vi "V003 - Variable DC Controller + Other Sensors.vi"() -> ()   [LabVIEW 2022 SP3]
uses:
  <vilib>/DAQmx/read.llb/DAQmx Read (Analog 1D DBL NChan 1Samp).vi
  <vilib>/DAQmx/create/channels.llb/DAQmx Create Channel (AI-Voltage-Basic).vi
  <vilib>/DAQmx/miscellaneous.llb/DAQmx Fill In Error Info.vi
panel:
  out "Case 0 Reached 2":bool
  out "Power Appl Ch3":bool
  in  "Appl CH3":bool
  out "Humidity":dbl(knob) scale=60.0..100.0
  out "Temperature":dbl(knob) scale=0.0..40.0
  out "Case 1 reached":bool
  out "CH2 Appl":bool
  in  "Appl CH2":bool
  out "Power On 3":bool
  out "Power On 2":bool
  in  "Turn On CH3":bool
  in  "Turn On CH2":bool
  out "Case 2  Reached":bool
  out "Case 1 Reached":bool
  in  "Numeric Controller Sub":dbl format="%#_1g"
  out "Power On":bool
  in  "Turn On CH1":bool
  out "Case 0 Reached":bool
  out "Connected":bool
  in  "VISA resource name":refnum<visa-resource-name>
  in  "Connect":bool
  in  "Numeric Controller Main":dbl
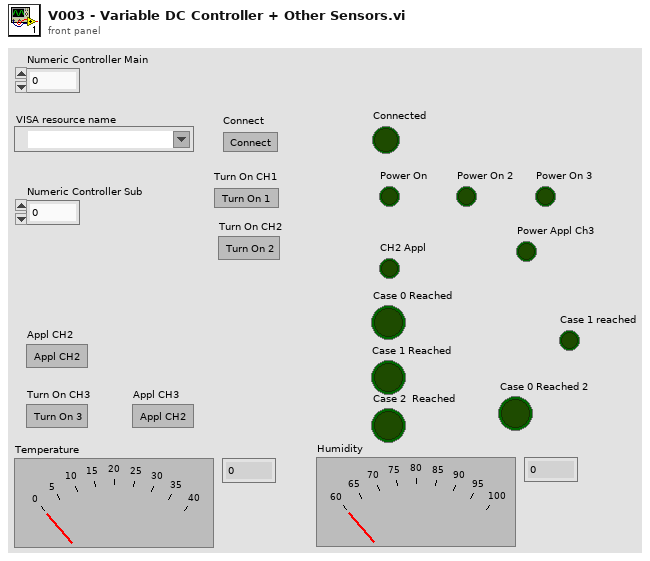
[diagram p1: front panel]
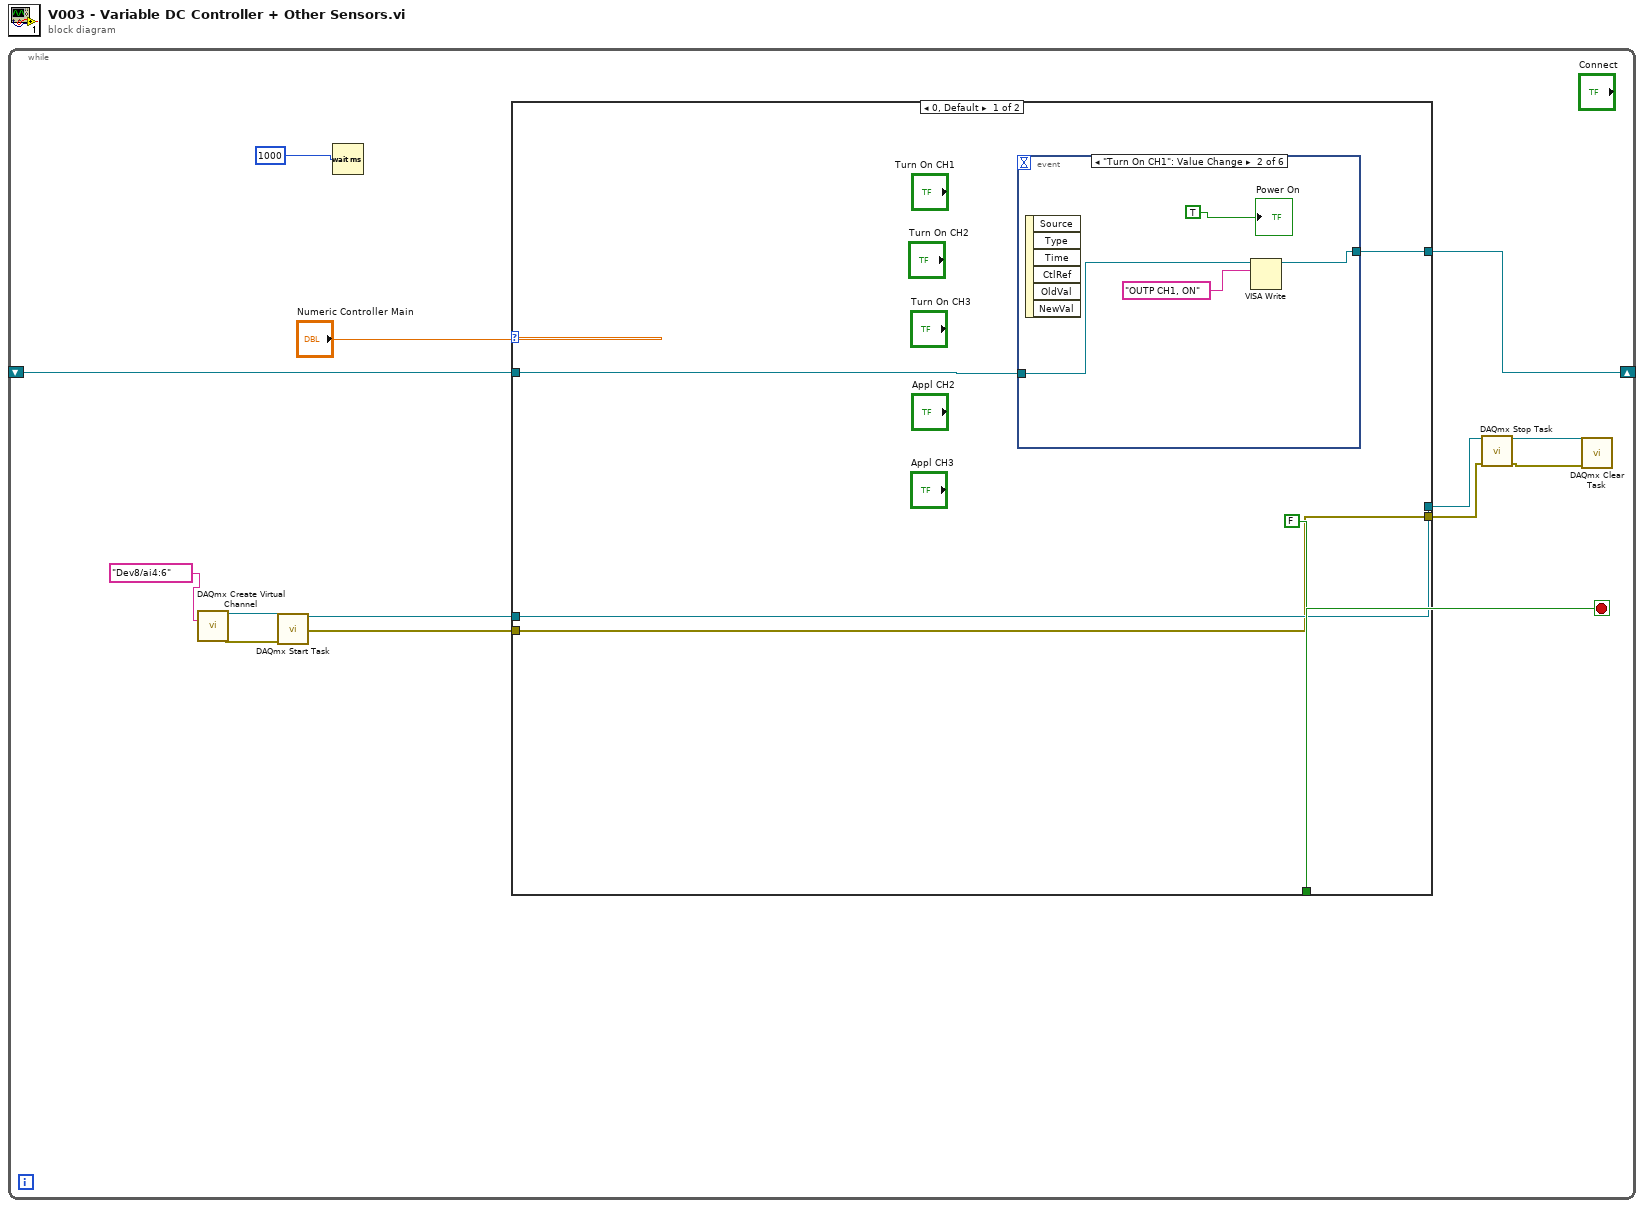
[diagram p0: block diagram]
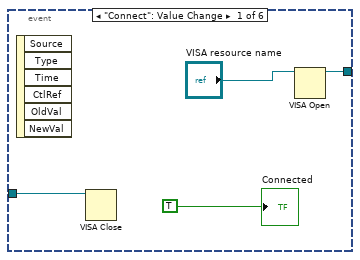
[diagram p2: hidden frame]
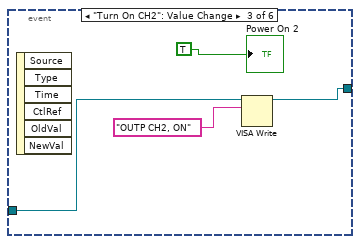
[diagram p3: hidden frame]
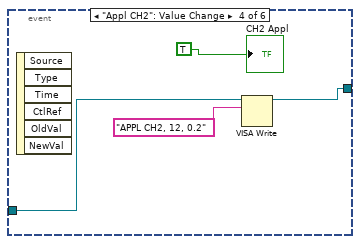
[diagram p4: hidden frame]
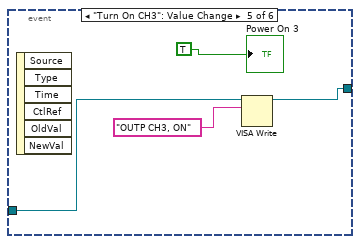
[diagram p5: hidden frame]
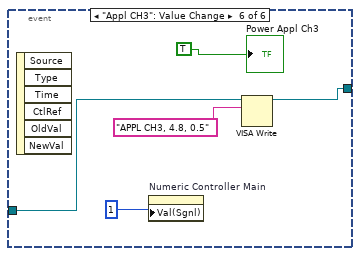
[diagram p6: hidden frame]
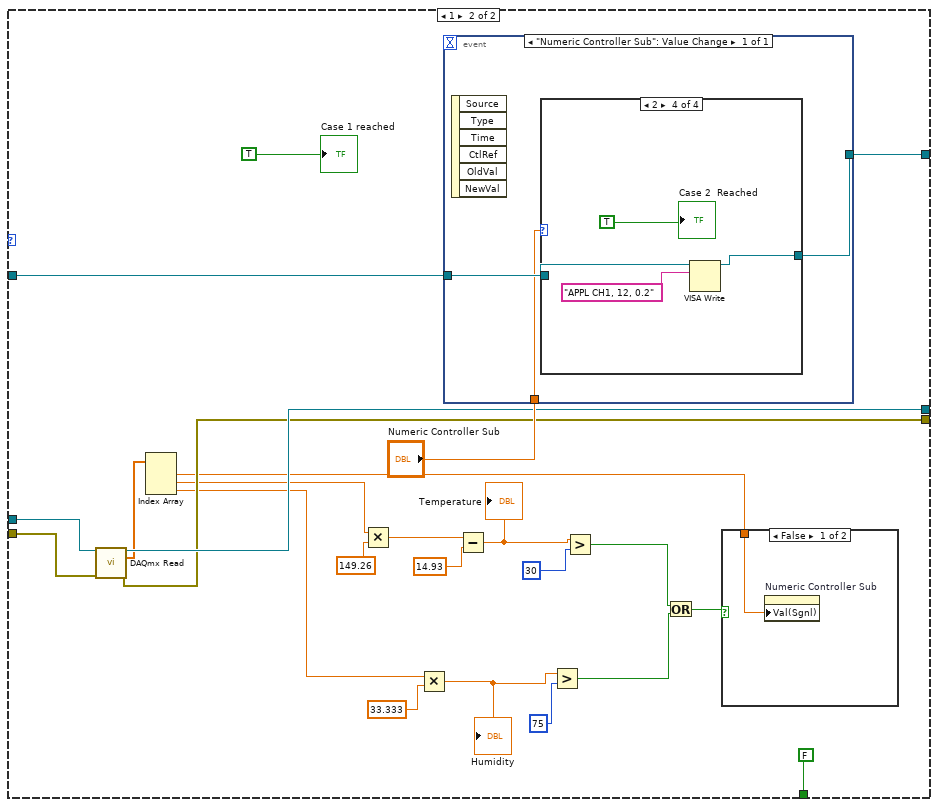
[diagram p7: hidden frame]
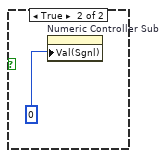
[diagram p8: hidden frame]
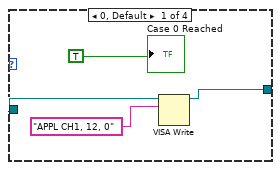
[diagram p9: hidden frame]
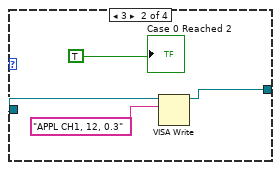
[diagram p10: hidden frame]
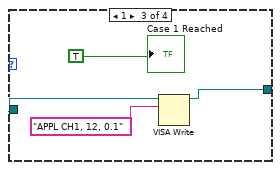
[diagram p11: hidden frame]
diagram:
  n1 = while {
    shift-right: [w13] -> _
    shift-left: _ -> [w14]
    stop <- w12 stop-if-true
    n2 = call-poly <vilib>:"DAQmx Create Virtual Channel.vi"("physical channels"=tag "Dev8/ai4:6") -> ("task out"=w10:refnum<k21>, "error out"=w6:errorcluster)  [unwired: 13 in]
    n3 = call <vilib>:"DAQmx Start Task.vi"("task/channels in"=w10, "error in"=w6) -> ("task out"=w8:refnum<k21>, "error out"=w7:errorcluster)  [unwired: 12 in]
    n4 = Wait (ms)(milliseconds to wait=1000) -> ()  [unwired: 1 out]
    n5 = case shown="0, Default" "Numeric Controller Main" {
      tunnel: w14 -> [w19 w66]
      tunnel: [w18 w67] -> w13
      tunnel: [FALSE FALSE] -> w12
      tunnel: w8 -> [w16 w64]
      tunnel: w7 -> [w15 w62]
      tunnel: [w16 w61] -> w2
      tunnel: [w15 w60] -> w1
      frame 0, Default {
        n6 = event shown="[1] \"Turn On CH1\": Value Change" {
          selector: _ -> [_ _ _ _ _ _]
          dyn-events: _ -> [_ _ _ _ _ _]
          timeout: _ -> [_ _ _ _ _ _]
          tunnel: w19 -> [w23 w26 w30 w34 w38 w43]
          tunnel: [w22 w25 w29 w33 w37 w42] -> w18
          event "Connect": Value Change {
            n7 = event-data() -> ()  [unwired: 1 in, 6 out]
            n8 = VISA Close(VISA resource name=w23) -> ()  [unwired: 1 in, 1 out]
            n9 = VISA Open(VISA resource name="VISA resource name") -> (VISA resource name=w22:refnum<visa-resource-name>)  [unwired: 4 in, 1 out]
            "Connected" <- TRUE
          }
          event "Turn On CH1": Value Change {
            n10 = event-data() -> ()  [unwired: 1 in, 6 out]
            n11 = VISA Write(VISA resource name=w26, write buffer="OUTP CH1, ON") -> (VISA resource name out=w25:refnum<visa-resource-name>)  [unwired: 1 in, 2 out]
            "Power On" <- TRUE
          }
          event "Turn On CH2": Value Change {
            n12 = event-data() -> ()  [unwired: 1 in, 6 out]
            n13 = VISA Write(VISA resource name=w30, write buffer="OUTP CH2, ON") -> (VISA resource name out=w29:refnum<visa-resource-name>)  [unwired: 1 in, 2 out]
            "Power On 2" <- TRUE
          }
          event "Appl CH2": Value Change {
            n14 = event-data() -> ()  [unwired: 1 in, 6 out]
            n15 = VISA Write(VISA resource name=w34, write buffer="APPL CH2, 12, 0.2") -> (VISA resource name out=w33:refnum<visa-resource-name>)  [unwired: 1 in, 2 out]
            "CH2 Appl" <- TRUE
          }
          event "Turn On CH3": Value Change {
            n16 = event-data() -> ()  [unwired: 1 in, 6 out]
            n17 = VISA Write(VISA resource name=w38, write buffer="OUTP CH3, ON") -> (VISA resource name out=w37:refnum<visa-resource-name>)  [unwired: 1 in, 2 out]
            "Power On 3" <- TRUE
          }
          event "Appl CH3": Value Change {
            n18 = event-data() -> ()  [unwired: 1 in, 6 out]
            n19 = property on="Numeric Controller Main" class="DigNum (strict)"("Val(Sgnl)"=1) -> ()  [unwired: 2 in, 2 out]
            n20 = VISA Write(VISA resource name=w43, write buffer="APPL CH3, 4.8, 0.5") -> (VISA resource name out=w42:refnum<visa-resource-name>)  [unwired: 1 in, 2 out]
            "Power Appl Ch3" <- TRUE
          }
        }
      }
      frame 1 {
        n21 = call-poly <vilib>:"DAQmx Read.vi"("task/channels in"=w64, "error in"=w62) -> ("task out"=w61:refnum<k21>, "data"=w59:dbl[], "error out"=w60:errorcluster)  [unwired: 11 in]
        n22 = Index Array(array=w59) -> (element #1=w45:dbl, element #2=w55:dbl, element #3=w54:dbl)  [unwired: 3 in]
        n23 = Multiply(x=w55, y=149.26) -> (x*y=w57:dbl)
        n24 = Multiply(x=w54, y=33.333) -> (x*y=w50:dbl)
        "Humidity" <- w50
        n25 = event shown="[0] \"Numeric Controller Sub\": Value Change" {
          selector: _ -> [_]
          dyn-events: _ -> [_]
          timeout: _ -> [_]
          tunnel: [w73] -> w67
          tunnel: w66 -> [w72]
          tunnel: "Numeric Controller Sub" -> [w71]
          event "Numeric Controller Sub": Value Change {
            n26 = event-data() -> ()  [unwired: 1 in, 6 out]
            n27 = case shown="2" w71 {
              tunnel: [w76 w80 w84 w88] -> w73
              tunnel: w72 -> [w75 w79 w83 w87]
              frame 0, Default {
                n28 = VISA Write(VISA resource name=w75, write buffer="APPL CH1, 12, 0") -> (VISA resource name out=w76:refnum<visa-resource-name>)  [unwired: 1 in, 2 out]
                "Case 0 Reached" <- TRUE
              }
              frame 3 {
                n29 = VISA Write(VISA resource name=w79, write buffer="APPL CH1, 12, 0.3") -> (VISA resource name out=w80:refnum<visa-resource-name>)  [unwired: 1 in, 2 out]
                "Case 0 Reached 2" <- TRUE
              }
              frame 1 {
                n30 = VISA Write(VISA resource name=w83, write buffer="APPL CH1, 12, 0.1") -> (VISA resource name out=w84:refnum<visa-resource-name>)  [unwired: 1 in, 2 out]
                "Case 1 Reached" <- TRUE
              }
              frame 2 {
                n31 = VISA Write(VISA resource name=w87, write buffer="APPL CH1, 12, 0.2") -> (VISA resource name out=w88:refnum<visa-resource-name>)  [unwired: 1 in, 2 out]
                "Case 2  Reached" <- TRUE
              }
            }
          }
        }
        n32 = Subtract(x=w57, y=14.93) -> (x-y=w52:dbl)
        "Temperature" <- w52
        n33 = Greater?(x=w50, y=75) -> (0:w47:bool)
        n34 = Greater?(x=w52, y=30) -> (0:w48:bool)
        n35 = Or(x=w48, y=w47) -> (x .or. y?=w46:bool)
        n36 = case shown="False" w46 {
          tunnel: w45 -> [w69 _]
          frame False {
            n37 = property on="Numeric Controller Sub" class="DigNum (strict)"("Val(Sgnl)"=w69) -> ()  [unwired: 2 in, 2 out]
          }
          frame True {
            n38 = property on="Numeric Controller Sub" class="DigNum (strict)"("Val(Sgnl)"=0) -> ()  [unwired: 2 in, 2 out]
          }
        }
        "Case 1 reached" <- TRUE
      }
    }
    n39 = call <vilib>:"DAQmx Stop Task.vi"("task/channels in"=w2, "error in"=w1) -> ("task out"=w4:refnum<k21>, "error out"=w3:errorcluster)  [unwired: 12 in]
    n40 = call <vilib>:"DAQmx Clear Task.vi"("task in"=w4, "error in"=w3) -> ()  [unwired: 13 in, 1 out]
  }
